vi "Binning.vi"() -> ()   [LabVIEW 2020]
uses:
  <vilib>/Analysis/2dsp.llb/Decimate (single shot, DBL).vi
  <vilib>/Analysis/NI_AALPro.lvlib
panel:
  out "min index(es)":i32[](array[numeric])
  out "min value":dbl
  out "max index(es)":i32[](array[numeric])
  out "max value":dbl
  in  "Decimated Array 2":dbl[][](array[numeric])
  out "Decimated Array":dbl[][](array[numeric])
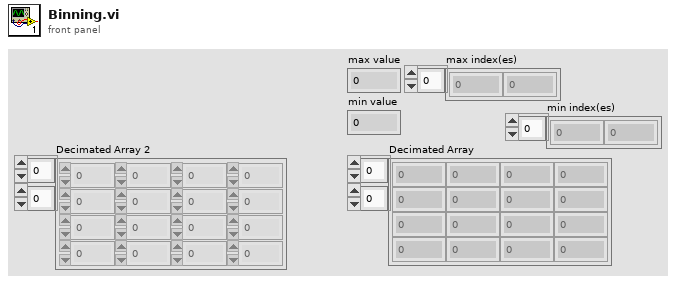
[diagram p1: front panel]
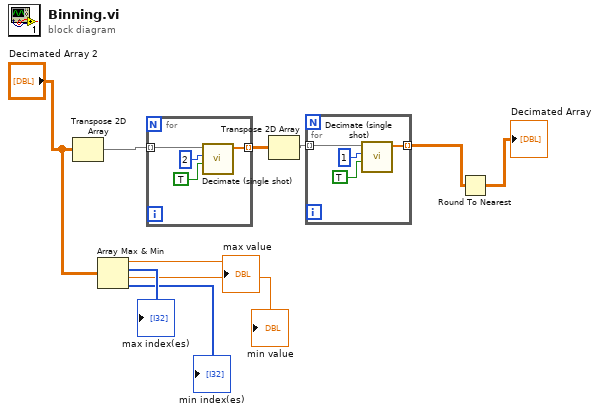
[diagram p0: block diagram]
diagram:
  n1 = Transpose 2D Array(2D array="Decimated Array 2") -> (transposed array=w10:dbl[][])
  n2 = Array Max & Min(array="Decimated Array 2") -> (max value=→"max value":dbl, max index (indices)=→"max index(es)":i32[], min value=→"min value":dbl, min index (indices)=→"min index(es)":i32[])
  n3 = for {
    tunnel: w10 -> [w12] mode=indexing
    tunnel: [w11] -> w9 mode=indexing
    n4 = call-poly <vilib>:"Decimate (single shot).vi"("averaging"=TRUE, "decimating factor"=2, "X"=w12) -> ("Decimated Array"=w11:dbl[])  [unwired: 7 in, 1 out]
  }
  n5 = Transpose 2D Array(2D array=w9) -> (transposed array=w8:dbl[][])
  n6 = for {
    tunnel: w8 -> [w16] mode=indexing
    tunnel: [w15] -> w2 mode=indexing
    n7 = call-poly <vilib>:"Decimate (single shot).vi"("averaging"=TRUE, "decimating factor"=1, "X"=w16) -> ("Decimated Array"=w15:dbl[])  [unwired: 7 in, 1 out]
  }
  n8 = Round To Nearest(number=w2) -> (nearest integer value=→"Decimated Array":dbl[][])
